vi "ocimode.vi"() -> ()   [LabVIEW 2012]
doc: "I. Description:\nThis example demonstrates how to acquire a continuous amount of data as a 2D array of Doubles in a DAQmx Base AI task. The acquired data is placed into a queue and passed from the producer loop to a consumer loop for processing. \n\nII. Instructions for Running:\nChoose the appropriate Physical Channel that corresponds to your device. Select the Maximum and Minimum Limits for acquisition. Select the Sample Rate for the Acquisition. Run the VI.\n\nIII. Block Diagram Steps:\n1. Create a DAQmx Base Task.\n2. Create an Analog Input Voltage Channel.\n3. Configure the AI Sample Clock.\n4. Start the Acquisition.\n5. Obtain a Queue for a 2D Array of Doubles.\n6. Read back the acquired data.\n7. Put the acquired data into the queue.\n8. Remove data from the queue.\n9. Release the queue.\n10. Stop the acquisition.\n11. Clear the DAQmx Base Task.\n12. Display any errors.\n\nIV. I/O Connections Overview:\nMake sure your signal input terminal matches the Physical Channel I/O Control. For further connection information, refer to your hardware reference manual."
uses:
  <vilib>/Utility/error.llb/DialogType.ctl
  <vilib>/_DAQmxBase/Internals/DAQmxBase Create Channel (AI-Voltage-Basic).vi
  <vilib>/_DAQmxBase/Internals/DAQmxBase Timing (Sample Clock).vi
  <vilib>/_DAQmxBase/Internals/DAQmxBase Read (Analog 2D DBL NChan NSamp).vi
panel:
  in  "DAQmx Physical Channel":tag
  out "Queue Size":i32(slide) scale=0.0..10.0
  out "ProdStopped":bool
  out "Data":dbl[][](graph)
  in  "Minimum Value":dbl=-10.0 format="%0.2f"
  in  "Maximum Value":dbl=10.0 format="%0.2f"
  in  "stop":bool
  in  "Sample Rate":dbl=10000.0 caption="Sample Rate (Hz)" format="%0.2f"
  # "For instructions, select Help>>Show Context Help"
  # "Channel Parameters"
  # "Timing Parameters"
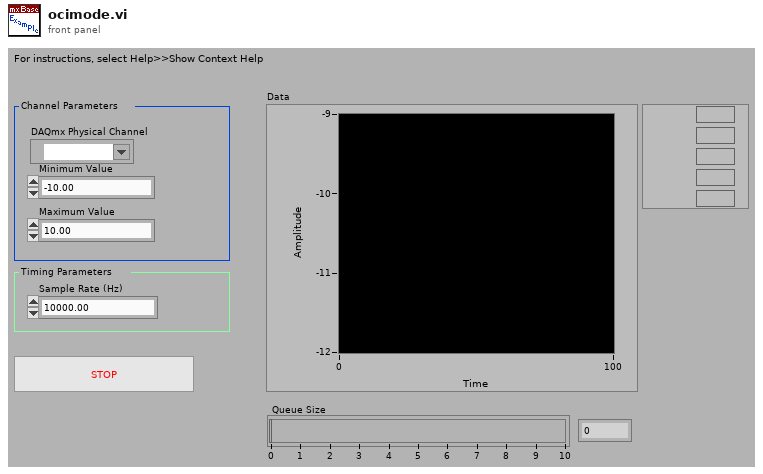
[diagram p1: front panel]
types:
  T1 = typedef "DialogType.ctl" = u16
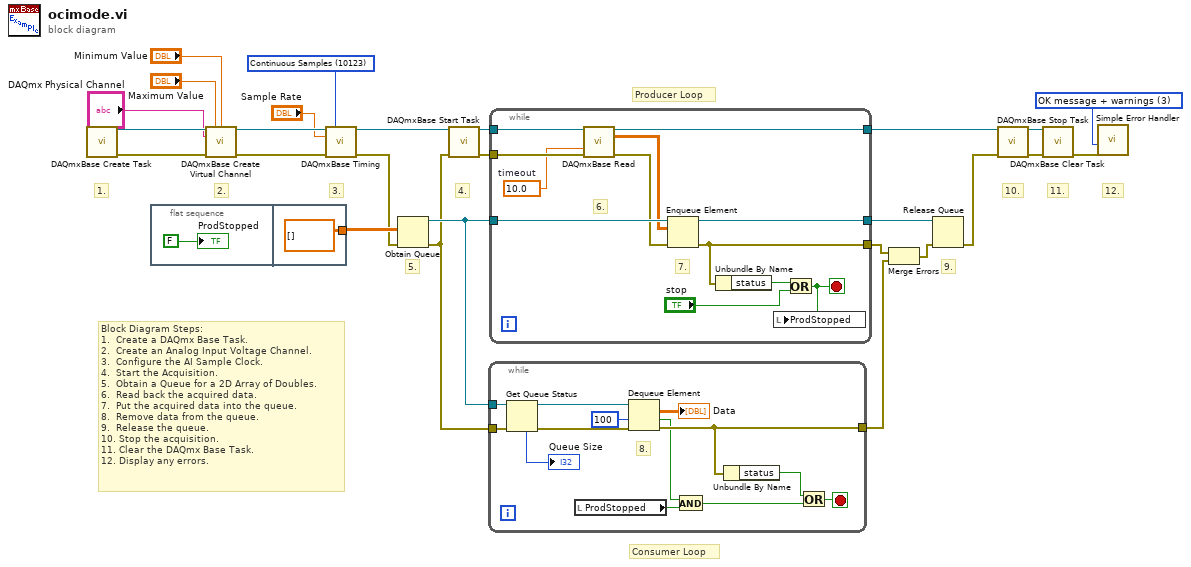
[diagram p0: block diagram]
diagram:
  w26 = T1 3 items=["no dialog", "OK message", "continue or stop message", "OK message + warnings", "continue/stop + warnings"] ("type of dialog (OK msg:1)")
  w16 = 10123 items=["Finite Samples"=10178, "Continuous Samples"=10123] ("sample mode")
  # "Consumer Loop"
  # "Producer Loop"
  # "Block Diagram Steps:\n1.  Create a DAQmx Base Task.\n2.  Create an Analog Input Voltage Channel.\n3.  Configure the AI Sample Clock.\n4.  Start the Acquisition.\n5.  Obtain a Queue for a 2D Array of Doubles.\n6.  Read back the acquired data.\n7.  Put the acquired data into the queue.\n8.  Remove data from the queue.\n9.  Release the queue.\n10. Stop the acquisition.\n11. Clear the DAQmx Base Task.\n12. Display any errors."
  # "12."
  # "11."
  # "10."
  # "9."
  # "5."
  # "4."
  # "3."
  # "2."
  # "1."
  n1 = call <vilib>:"DAQmxBase Create Task.vi"() -> ("task out"=w24:refnum<k21>, "error out"=w25:errorcluster)  [unwired: 5 in, 9 out]
  n2 = flat-sequence {
    tunnel: [dbl[][] []] -> w8
    frame #0 {
      "ProdStopped" <- FALSE ("ProdStopped")
    }
    frame #1 {
    }
  }
  n3 = call-poly <vilib>:"DAQmxBase Create Virtual Channel.vi"("task in"=w24, "maximum value"="Maximum Value", "minimum value"="Minimum Value", "physical channels"="DAQmx Physical Channel", "error in"=w25) -> ("task out"=w22:refnum<k21>, "error out"=w23:errorcluster)  [unwired: 4 in, 5 out]
  n4 = call-poly <vilib>:"DAQmxBase Timing.vi"("task/channels in"=w22, "sample mode"=w16, "rate"="Sample Rate", "error in"=w23) -> ("task out"=w21:refnum<k21>, "error out"=w4:errorcluster)  [unwired: 3 in, 7 out]
  n5 = Obtain Queue(element data type=w8, error in (no error)=w4) -> (queue out=w9:refnum<queue>, error out=w3:errorcluster)  [unwired: 2 in, 2 out]
  n6 = call <vilib>:"DAQmxBase Start Task.vi"("task/channels in"=w21, "error in"=w3) -> ("task out"=w12:refnum<k21>, "error out"=w11:errorcluster)  [unwired: 12 out]
  n7 = while {
    tunnel: w9 -> [w33]
    tunnel: w3 -> [w30]
    tunnel: [w38] -> w5
    stop <- w41 stop-if-true
    # "8."
    n8 = Get Queue Status(queue=w33, error in (no error)=w30) -> (queue out=w32:refnum<queue>, error out=w31:errorcluster, # elements in queue=→"Queue Size":i32)  [unwired: 6 out]
    n9 = local read "ProdStopped"() -> (w34:bool)
    n10 = Dequeue Element(queue=w32, timeout in ms (-1)=100, error in (no error)=w31) -> (element=→"Data":dbl[][], timed out?=w36:bool, error out=w38:errorcluster)  [unwired: 1 out]
    n11 = And(x=w36, y=w34) -> (x .and. y?=w35:bool)
    n12 = Unbundle By Name(w38) -> ("status"=w39:bool)
    n13 = Or(x=w39, y=w35) -> (x .or. y?=w41:bool)
  }
  n14 = while {
    tunnel: [w53] -> w20
    tunnel: w12 -> [w52]
    tunnel: w11 -> [w51]
    tunnel: w9 -> [w49]
    tunnel: [w48] -> w10
    tunnel: [w46] -> w6
    stop <- w42 stop-if-true
    w50 = 10.0  # timeout
    # "7."
    # "6."
    n15 = call-poly <vilib>:"DAQmxBase Read.vi"("task/channels in"=w52, "timeout"=w50, "error in"=w51) -> ("task out"=w53:refnum<k21>, "data"=w47:dbl[][], "error out"=w44:errorcluster)  [unwired: 1 in, 9 out]
    n16 = Enqueue Element(queue=w49, element=w47, error in (no error)=w44) -> (queue out=w48:refnum<queue>, error out=w46:errorcluster)  [unwired: 2 out]
    n17 = Unbundle By Name(w46) -> ("status"=w45:bool)
    n18 = Or(x=w45, y="stop") -> (x .or. y?=w42:bool)
    n19 = local write "ProdStopped"(w42) -> ()
  }
  n20 = Merge Errors(w6, w5) -> (w7:errorcluster)
  n21 = Release Queue(queue=w10, error in (no error)=w7) -> (error out=w2:errorcluster)  [unwired: 3 out]
  n22 = call <vilib>:"DAQmxBase Stop Task.vi"("task/channels in"=w20, "error in"=w2) -> ("task out"=w18:refnum<k21>, "error out"=w19:errorcluster)  [unwired: 12 out]
  n23 = call <vilib>:"DAQmxBase Clear Task.vi"("task in"=w18, "error in"=w19) -> ("error out"=w17:errorcluster)  [unwired: 13 out]
  n24 = call <vilib>:"Simple Error Handler.vi"("type of dialog (OK msg:1)"=w26, "error in (no error)"=w17) -> ()  [unwired: 8 out]
